vi "Save Results to TDMS.vi"(1 "measurement configuration":T1={"Mode of operation"=enum."Perform measurement", "DUT setup time"=1.0, "Nominal output voltage"=3.3, "Source pin name"="", "Source sense"=1009, "Source current limit"=25.0, "Source voltage level"=12.0, "Source transient response"=1042, "Source voltage gain bandwidth"=2000.0, "Source voltage compensation frequency"=3530.0, "Source voltage pole-zero ratio"=2.0, "Load pin name"="", "Load sense"=1009, "Load voltage limit range"=6.0, "Load current level range"=40.0, "Load sample rate"=1800000.0, "Load current set point 1"=4.0, "Load current set point 2"=14.0, "Load current delay t1"=0.001, "Load current pulse duration"=0.001, "Load current delay t2"=0.001, "Load current rising slew rate"=24.0, "Load current falling slew rate"=24.0, "Load transient response"=1042, "Load current gain bandwidth"=14000.0, "Load current compensation frequency"=180000.0, "Load current pole-zero ratio"=0.3, "Pin Names for Scope"=[], "vertical range"=[], "vertical offset"=[], "probe attenuation"=[], "vertical coupling"=[], "input impedance"=[], "max input frequency"=[], "min record length"=[], "channel enabled"=[], "enforce realtime"=[], "reference position"=[], "min sample rate"=[]} {"input impedance" items=["1 mega ohm"=0, "50 ohms"=2]; "vertical coupling" items=["AC", "DC", "Ground"]; "Load transient response" items=["Slow"=1041, "Normal"=1038, "Fast"=1039, "Custom"=1042]; "Load current falling slew rate" format="%#_6p"; "Load current rising slew rate" format="%#_6p"; "Load current level range" format="%#_6p"; "Load voltage limit range" format="%#_6p"; "Load sense" items=["Local"=1008, "Remote"=1009]; "Source transient response" items=["Slow"=1041, "Normal"=1038, "Fast"=1039, "Custom"=1042]; "Source sense" items=["Local"=1008, "Remote"=1009]; "Nominal output voltage" format="%#_6pV"}, 3 "measurement results":T3, 4 "Scope waveforms":waveform(dbl)[](array[waveform]), 5 "error in (no error)":errorcluster) -> (19 "error out":errorcluster)   [LabVIEW 2021, in "Load Transient Response with Pin Map.lvlib"]
uses:
  Load Transient Response with Pin Map.lvlib
  <vilib>/Utility/sysdir.llb/System Directory Type.ctl
  Measurement Results.ctl
  <instrlib>/niScope/Controls/niScope vertical coupling.ctl
  Measurement Configuration.ctl
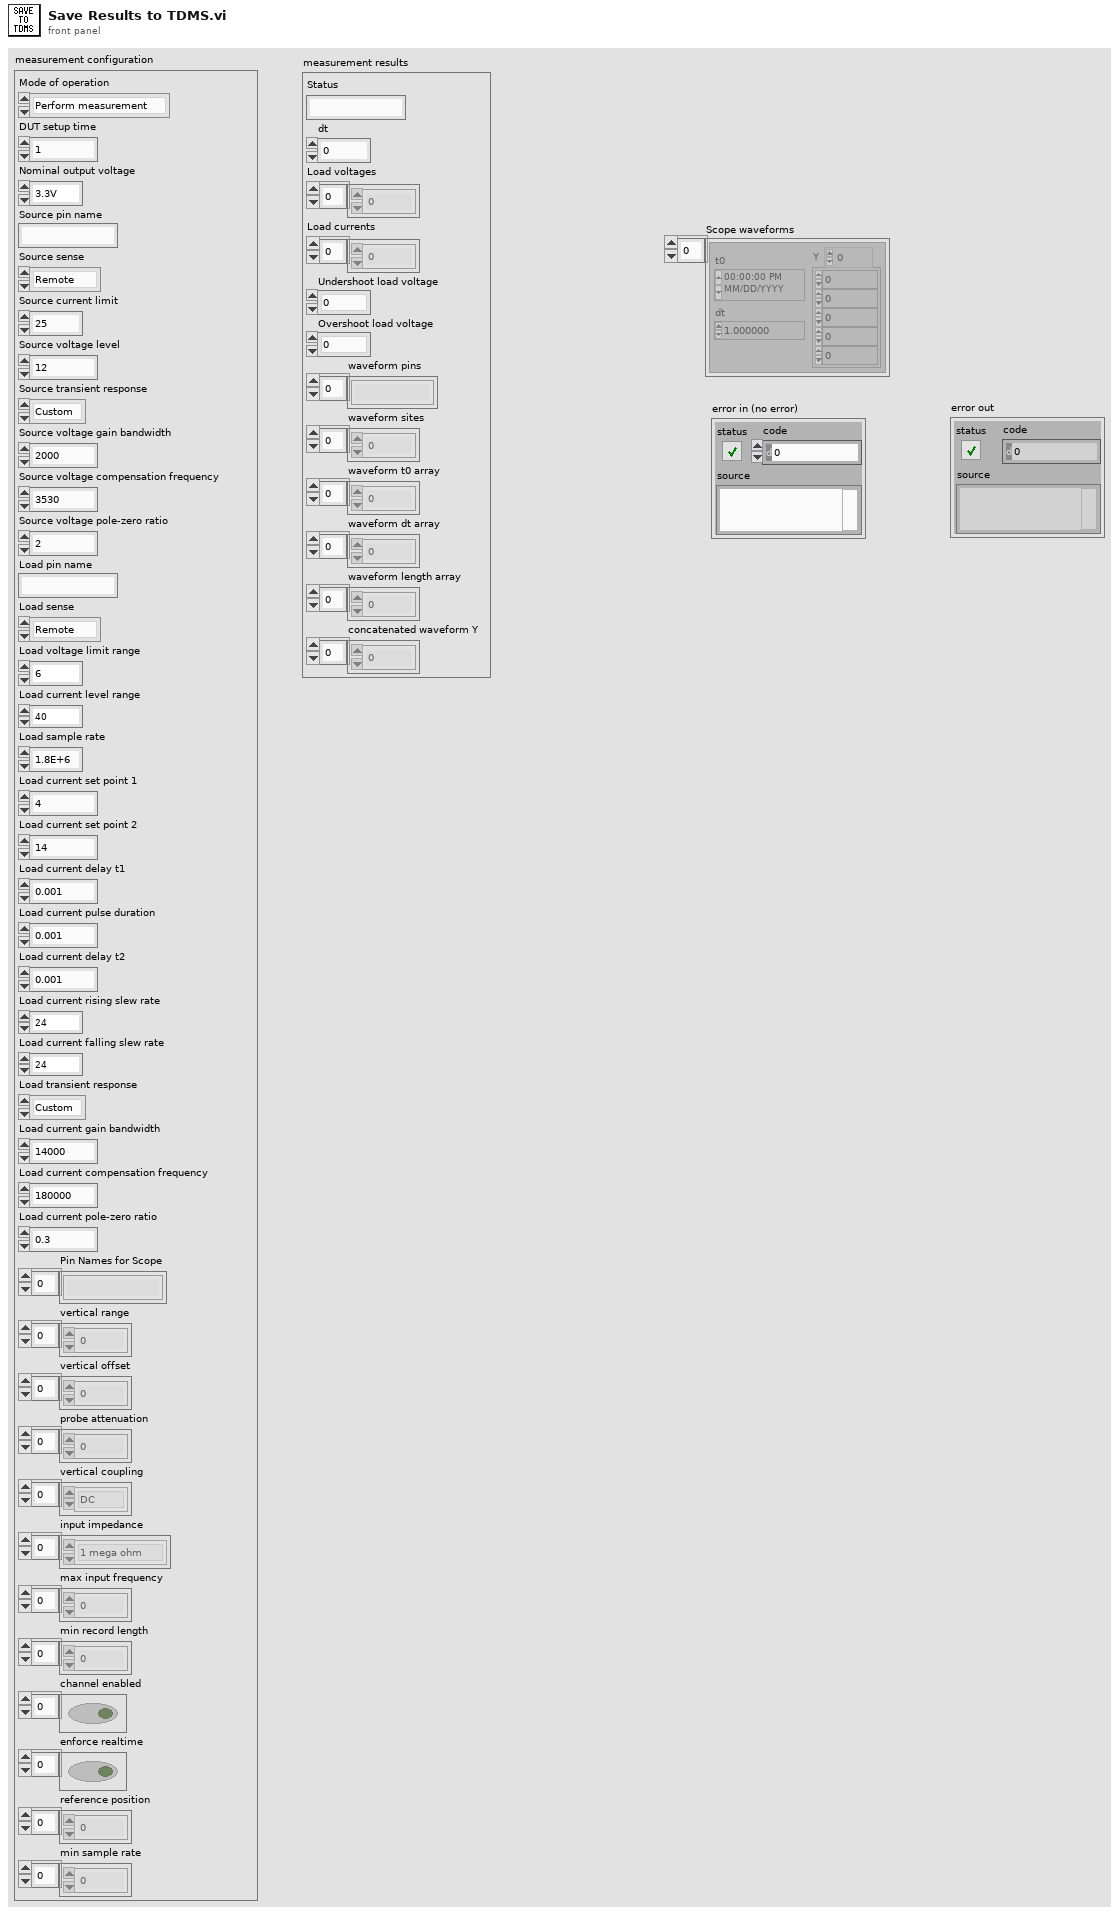
[diagram p1: front panel]
types:
  T1 = typedef "Load Transient Response with Pin Map.lvlib/Measurement Configuration.ctl" = cluster{"Mode of operation":enum32{"Power on the DUT", "Perform measurement", "Power off the DUT"}, "DUT setup time":dbl, "Nominal output voltage":dbl, "Source pin name":string, "Source sense":i32, "Source current limit":dbl, "Source voltage level":dbl, "Source transient response":i32, "Source voltage gain bandwidth":dbl, "Source voltage compensation frequency":dbl, "Source voltage pole-zero ratio":dbl, "Load pin name":string, "Load sense":i32, "Load voltage limit range":dbl, "Load current level range":dbl, "Load sample rate":dbl, "Load current set point 1":dbl, "Load current set point 2":dbl, "Load current delay t1":dbl, "Load current pulse duration":dbl, "Load current delay t2":dbl, "Load current rising slew rate":dbl, "Load current falling slew rate":dbl, "Load transient response":i32, "Load current gain bandwidth":dbl, "Load current compensation frequency":dbl, "Load current pole-zero ratio":dbl, "Pin Names for Scope":string[], "vertical range":dbl[], "vertical offset":dbl[], "probe attenuation":dbl[], "vertical coupling":T2[], "input impedance":u32[], "max input frequency":dbl[], "min record length":i32[], "channel enabled":bool[], "enforce realtime":bool[], "reference position":dbl[], "min sample rate":dbl[]}
  T2 = typedef "niScope vertical coupling.ctl" = i32
  T3 = typedef "Load Transient Response with Pin Map.lvlib/Measurement Results.ctl" = cluster{"Status":string, "dt":dbl, "Load voltages":dbl[], "Load currents":dbl[], "Undershoot load voltage":dbl, "Overshoot load voltage":dbl, "waveform pins":string[], "waveform sites":i32[], "waveform t0 array":dbl[], "waveform dt array":dbl[], "waveform length array":i32[], "concatenated waveform Y":dbl[]}
  T4 = typedef "System Directory Type.ctl" = i32
  T5 = enum16{"open", "open or create", "create or replace", "create", "open (read-only)"}
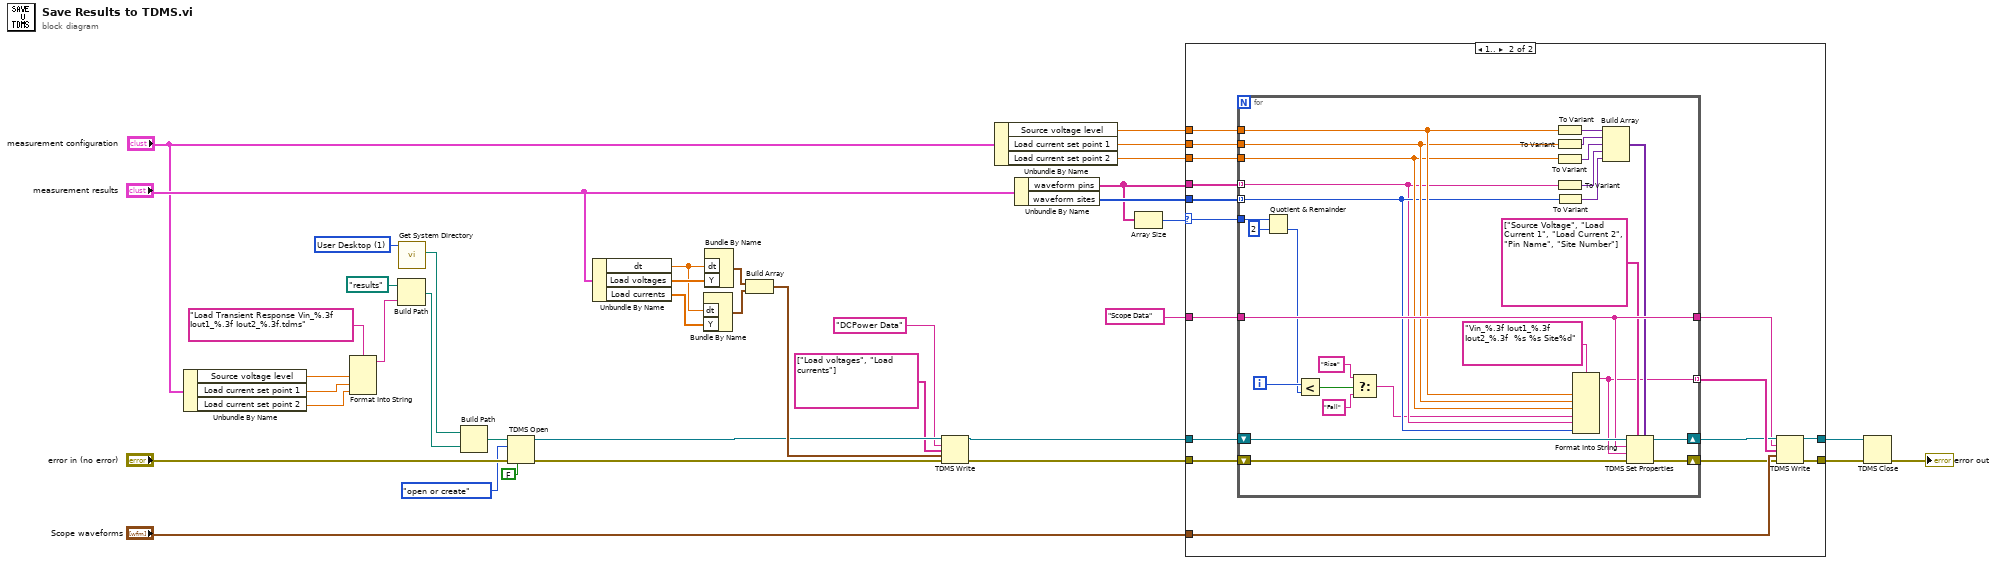
[diagram p0: block diagram]
diagram:
  w2 = T4 1 items=["User Home"=0, "User Desktop"=1, "User Documents"=2, "User Application Data"=3, "User Preferences"=4, "User Temporary"=5, "Public Documents"=6, "Public Application Data"=7, "Public Preferences"=8, "Public Cache"=13, "System Core Libraries"=9, "System Installed Libraries"=10, "Application Files"=11, "Boot Volume Root"=12] ("system directory type")
  n1 = Unbundle By Name("measurement configuration") -> ("Source voltage level"=w14:dbl, "Load current set point 1"=w13:dbl, "Load current set point 2"=w12:dbl)
  n2 = Format Into String(format string="Load Transient Response Vin_%.3f Iout1_%.3f Iout2_%.3f.tdms", w14, w13, w12) -> (resulting string=w10:string)  [unwired: 2 in, 1 out]
  n3 = Build Path(base path=path "results", name or relative path=w10) -> (appended path=w9:path)
  n4 = call <vilib>:"Get System Directory.vi"("system directory type"=w2) -> ("system directory"=w1:path)  [unwired: 10 in]
  n5 = Build Path(base path=w1, name or relative path=w9) -> (appended path=w28:path)
  n6 = TDMS Open(6:FALSE ("disable buffering? (T)"), 8:"error in (no error)", 10:T5."open or create" ("operation (0:open)"), 11:w28) -> (0:w7:errorcluster, 3:w8:refnum<k34>)  [unwired: 3 in]
  n7 = Unbundle By Name("measurement results") -> ("dt"=w21:dbl, "Load voltages"=w23:dbl[], "Load currents"=w22:dbl[])
  n8 = Bundle By Name("dt"=w21, "Y"=w22) -> (w18:waveform(dbl))  [unwired: 1 in]
  n9 = Bundle By Name("dt"=w21, "Y"=w23) -> (w19:waveform(dbl))  [unwired: 1 in]
  n10 = Build Array(w19, w18) -> (w17:waveform(dbl)[])
  n11 = TDMS Write(0:w8, 5:"DCPower Data" ("group name in (Untitled)"), 7:string[] ["Load voltages", "Load currents"], 9:w17, 11:w7) -> (4:w4:refnum<k34>, 15:w3:errorcluster)  [unwired: 1 in, 2 out]
  n12 = Unbundle By Name("measurement configuration") -> ("Source voltage level"=w33:dbl, "Load current set point 1"=w35:dbl, "Load current set point 2"=w20:dbl)
  n13 = Unbundle By Name("measurement results") -> ("waveform pins"=w25:string[], "waveform sites"=w26:i32[])
  n14 = Array Size(array=w25) -> (size(s)=w27:i32)
  n15 = case shown="1.." w27 {
    selector: w27 -> [_ w41]
    tunnel: "Scope waveforms" -> [_ w56]
    tunnel: w35 -> [_ w55]
    tunnel: w25 -> [_ w53]
    tunnel: "Scope Data" ("group name in (Untitled)") -> [_ w50]
    tunnel: w33 -> [_ w48]
    tunnel: w3 -> [w40 w47]
    tunnel: w4 -> [w39 w46]
    tunnel: [w40 w45] -> w30
    tunnel: [w39 w44] -> w29
    tunnel: w26 -> [_ w43]
    tunnel: w20 -> [_ w42]
    frame 0, Default {
      # "Do nothing if Pin Names are emply."
    }
    frame 1.. {
      n16 = for {
        tunnel: w48 -> [w76]
        tunnel: w55 -> [w75]
        tunnel: w53 -> [w65] mode=indexing
        tunnel: [w71] -> w54 mode=indexing
        shift-right: [w81] -> w52
        shift-left: w46 -> [w82]
        shift-right: [w79] -> w51
        shift-left: w47 -> [w80]
        tunnel: w50 -> [w78]
        tunnel: [w78] -> w49
        tunnel: w43 -> [w66] mode=indexing
        tunnel: w42 -> [w67]
        tunnel: w41 -> [w64]
        i -> [w62]
        n17 = Quotient & Remainder(x=w64, y=2) -> (floor(x/y)=w61:i32)  [unwired: 1 out]
        n18 = Less?(x=w62, y=w61) -> (x < y?=w58:bool)
        n19 = Select(t="Rise", s=w58, f="Fall") -> (s? t:f=w57:string)
        n20 = To Variant(anything=w76) -> (Variant=w74:variant)
        n21 = To Variant(anything=w75) -> (Variant=w73:variant)
        n22 = To Variant(anything=w67) -> (Variant=w68:variant)
        n23 = To Variant(anything=w65) -> (Variant=w70:variant)
        n24 = To Variant(anything=w66) -> (Variant=w69:variant)
        n25 = Format Into String(format string="Vin_%.3f Iout1_%.3f Iout2_%.3f  %s %s Site%d", w76, w75, w67, w57, w65, w66) -> (resulting string=w71:string)  [unwired: 2 in, 1 out]
        n26 = Build Array(w74, w73, w68, w70, w69) -> (w72:variant[])
        n27 = TDMS Set Properties(5:w72, 7:string[] ["Source Voltage", "Load Current 1", "Load Current 2", "Pin Name", "Site Number"] ("property names"), 8:w80, 9:w71, 10:w78, 11:w82) -> (0:w79:errorcluster, 3:w81:refnum<k34>)  [unwired: 2 out]
      }
      n28 = TDMS Write(0:w52, 5:w49, 7:w54, 9:w56, 11:w51) -> (4:w44:refnum<k34>, 15:w45:errorcluster)  [unwired: 1 in, 2 out]
    }
  }
  n29 = TDMS Close(8:w30, 11:w29) -> (0:→"error out":errorcluster)  [unwired: 1 out]
